vi "Lbs Or Kips.vi"(6 "Size":T1, 10 "Cartesian Force In":string[](array[string])=[" Fx (lb)", " Fy (lb)", " Fz (lb)", " Mx (lb*in)", " My (lb*in)", " Mz (lb*in)"]) -> (2 "Cartesian Force In Out":string[](array[string])=[" Fx (lb)", " Fy (lb)", " Fz (lb)", " Mx (lb*in)", " My (lb*in)", " Mz (lb*in)"])   [LabVIEW 2009]
uses:
  Data Access Objects/Metadata/LBCB Size.ctl
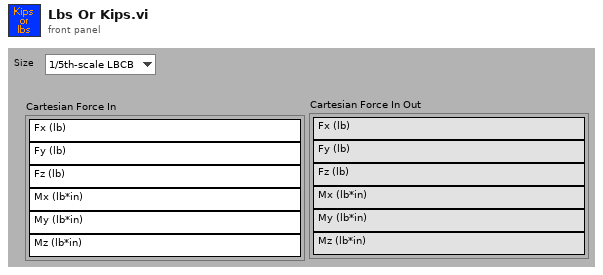
[diagram p1: front panel]
types:
  T1 = typedef "LBCB Size.ctl" = enum16{"1/5th-scale LBCB", "Full-scale LBCB", "Portable LBCB", "Mid-Scale LBCB"}
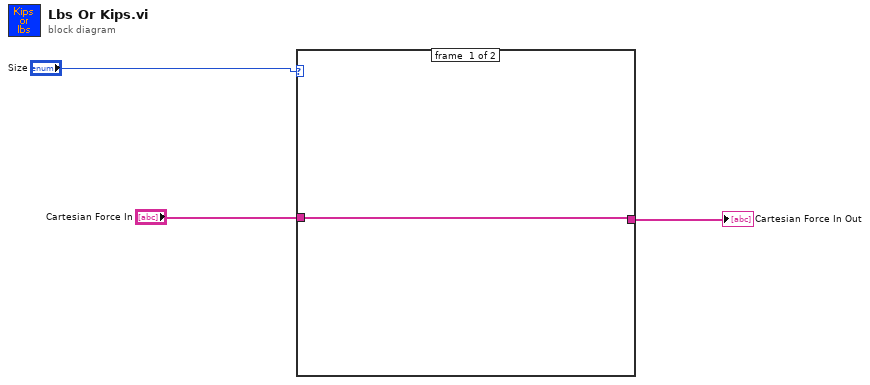
[diagram p0: block diagram]
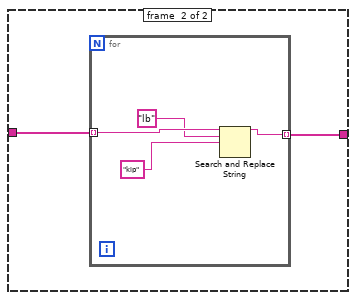
[diagram p2: hidden frame]
diagram:
  n1 = case shown="\"1/5th-scale LBCB\", Default" "Size" {
    tunnel: "Cartesian Force In" -> [w4 w6]
    tunnel: [w4 w5] -> w1
    frame #0 {
    }
    frame #1 {
      n2 = for {
        tunnel: w6 -> [w10] mode=indexing
        tunnel: [w7] -> w5 mode=indexing
        n3 = Search and Replace String(input string=w10, search string="lb", replace string="kip" ("replace string (\"\")")) -> (result string=w7:string)  [unwired: 5 in, 3 out]
      }
    }
  }
  "Cartesian Force In Out" <- w1
